vi "manual temp control.vi"(11 "error in":errorcluster, 13 "Normalized Power In (0-1)":dbl format="%.2f") -> (4 "power meas (0-1)":dbl format="%.2f", 8 "temp meas":dbl=26.795989484821064 format="%.2f", 15 "error out":errorcluster)   [LabVIEW 2014]
doc: "This vi manages the temperature measurement and power control\n\nPaul K Dixon\nPhysics 350\nPaul K Dixon"
panel:
  # "Manual Temperature Control"
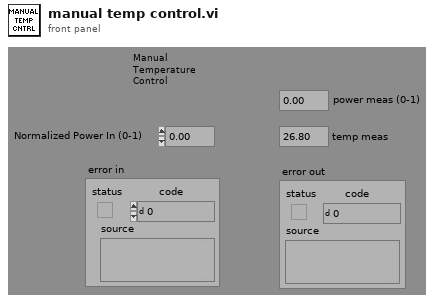
[diagram p1: front panel]
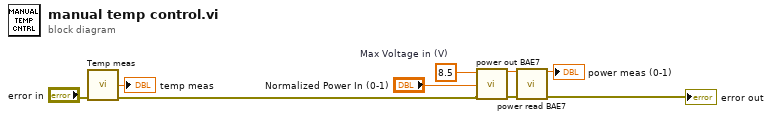
[diagram p0: block diagram]
diagram:
  w6 = 8.5  # Max Voltage in (V)
  n1 = call "Temp meas.vi"("error in"="error in") -> ("Temp (deg C)"=→"temp meas":dbl, "error out"=w5:errorcluster)  [unwired: 11 in, 2 out]
  n2 = call "power out BAE7.vi"("Max Voltage in (V)"=w6, "Normalized Power (0-1)"="Normalized Power In (0-1)", "error in (no error)"=w5) -> ("Max Voltage out (V)"=w4:dbl, "error out"=w3:errorcluster)  [unwired: 11 in]
  n3 = call "power read BAE7.vi"("Max Voltage in"=w4, "error in (no error)"=w3) -> ("normalized Power Read (0-1)"=→"power meas (0-1)":dbl, "error out"=→"error out":errorcluster)  [unwired: 12 in]
